vi "rescale intensity imaq image.vi"(2 "Image Dst":T1, 3 "Image in":T1) -> (0 "Maximal Value":sgl, 1 "Image Dst Out":T1)   [LabVIEW 2013]
uses:
  <vilib>/vision/Image Controls.llb/IMAQ Image.ctl
  <vilib>/vision/NI_Vision_Development_Module.lvlib
panel:
  out "error out":errorcluster
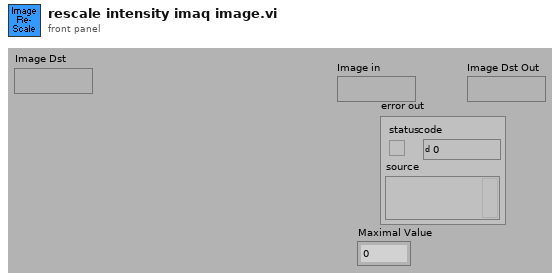
[diagram p1: front panel]
types:
  T1 = typedef "IMAQ Image.ctl" = refnum<image>
  T2 = cluster{"histogram":u32[], "Minimal Value":sgl, "Maximal Value":sgl, "Starting Value":sgl, "Interval Width":sgl, "Mean Value":sgl, "Standard  Variation":sgl, "Area (pixels)":i32}
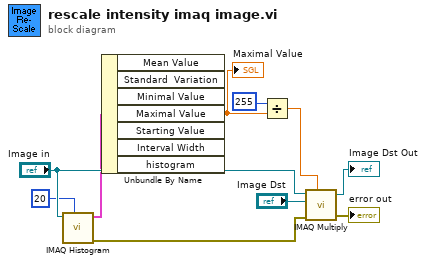
[diagram p0: block diagram]
diagram:
  n1 = call "IMAQ Histogram"("Number of Classes"=20, "Image"="Image in") -> ("error out"=w3:errorcluster, "Histogram Report"=w5:T2)  [unwired: 3 in, 5 out]
  n2 = Unbundle By Name(w5) -> ("Maximal Value"=w4:sgl)  [unwired: 6 out]
  "Maximal Value" <- w4
  n3 = Divide(x=255, y=w4) -> (x/y=w9:sgl)
  n4 = call "IMAQ Multiply"("Image Src A"="Image in", "Constant"=w9, "Image Dst"="Image Dst", "error in (no error)"=w3) -> ("Image Dst Out"=→"Image Dst Out":T1, "error out"=→"error out":errorcluster)  [unwired: 3 in]
